vi "Write Msg Input.vi"(10 "Msg Input":refnum<class "Msg Input.lvclass">, 11 "Stop Msg in":refnum<class "Stop Msg.lvclass">) -> (3 "Stop Msg out":refnum<class "Stop Msg.lvclass">)   [LabVIEW 2020, in "jettl.lvlib" / "Stop jettl Msg.lvlib" / "Stop Msg.lvlib" / "Stop Msg.lvclass"]
uses:
  Stop Msg.lvclass
  Msg Input/Msg Input.lvclass
  Stop Msg.lvclass/Stop Msg.ctl
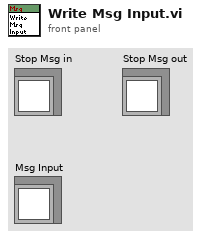
[diagram p1: front panel]
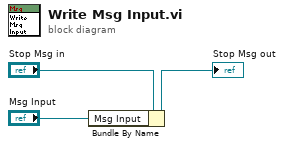
[diagram p0: block diagram]
diagram:
  n1 = Bundle By Name(cluster="Stop Msg in", "Msg Input"="Msg Input") -> (→"Stop Msg out":refnum<class "Stop Msg.lvclass">)
